vi "Set Valve.vi"(8 "error in (no error)":errorcluster, 10 "Open/Close":bool=TRUE, 11 "Freezer in":refnum<class "Freezer.lvclass">) -> (0 "error out":errorcluster, 3 "Freezer out":refnum<class "Freezer.lvclass">)   [LabVIEW 2015, in "cRIO-Carbondioxide.lvlib" / "CO2-Actor.lvlib" / "Freezer.lvclass"]
uses:
  Freezer.lvclass
  Freezer.lvclass/Freezer.ctl
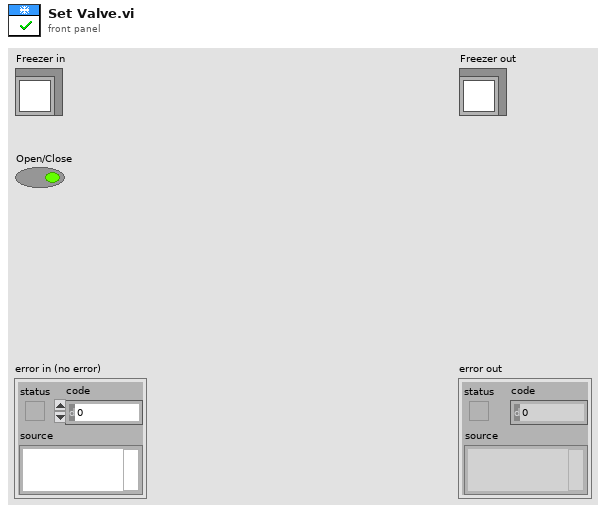
[diagram p1: front panel]
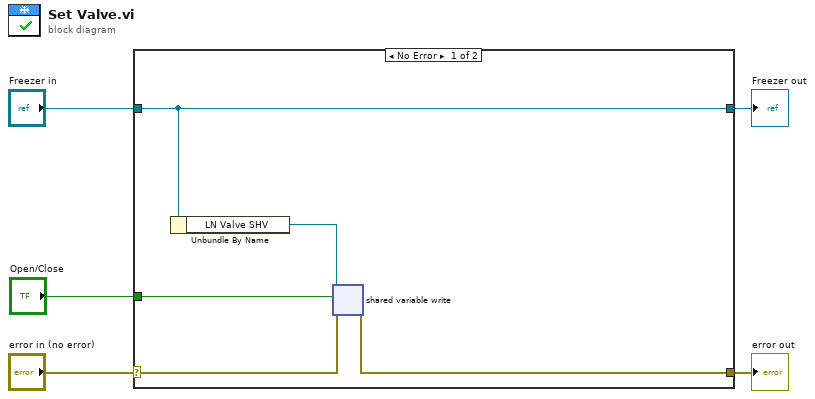
[diagram p0: block diagram]
diagram:
  n1 = case shown="No Error" "error in (no error)" {
    selector: "error in (no error)" -> [w8 w12]
    tunnel: [w7 w12] -> w4
    tunnel: [w10 w11] -> w2
    tunnel: "Freezer in" -> [w10 w11]
    tunnel: "Open/Close" -> [w6 _]
    frame No Error {
      n2 = Unbundle By Name(w10) -> ("LN Valve SHV"=w9:refnum<k21>)
      n3 = shared-variable-write(w9, w8, w6) -> (w7:errorcluster)  [unwired: 1 out]
    }
    frame Error {
    }
  }
  "error out" <- w4
  "Freezer out" <- w2
